vi "TeardownAfterStart.vi"(6 "Error":errorcluster, 7 "Actor":refnum<class "Actor.lvclass">, 11 "UnheardMessages":refnum<class "Message.lvclass">[](array[class])) -> (5 "Actor":refnum<class "Actor.lvclass">)   [LabVIEW 2020, in "jettl.lvlib" / "Actor.lvclass"]
uses:
  Actor.lvclass
  Message/Message.lvclass
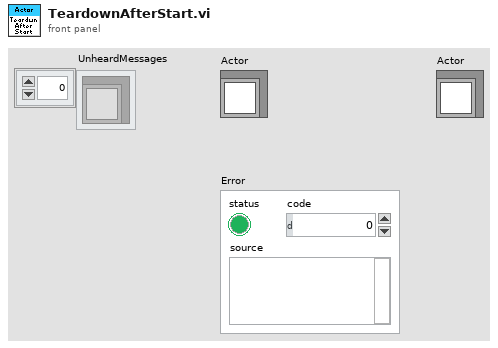
[diagram p1: front panel]
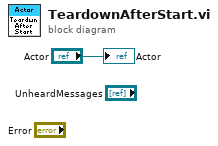
[diagram p0: block diagram]
diagram:
  "Actor" <- "Actor"
